vi "Configure Specific Limit Test.vi"(0 "VISA resource name":refnum<visa-resource-name>, 1 "Enable Limit Test  (T:Enable)":bool=TRUE, 5 "Limit Test Number (2)":u16=2, 7 "Low Limit (0)":dbl, 9 "High Limit (1)":dbl=1.0, 11 "error in (no error)":errorcluster, 12 "I/O Output Settings":T1) -> (4 "VISA resource name out":refnum<visa-resource-name>, 15 "error out":errorcluster)   [LabVIEW 2015, in "VIPM2.lvlib" / "Keithley 24XX.lvlib"]
doc: "Configures limit testing settings, such as the source of the tested value, binning, and I/O settings."
uses:
  Keithley 24XX.lvlib
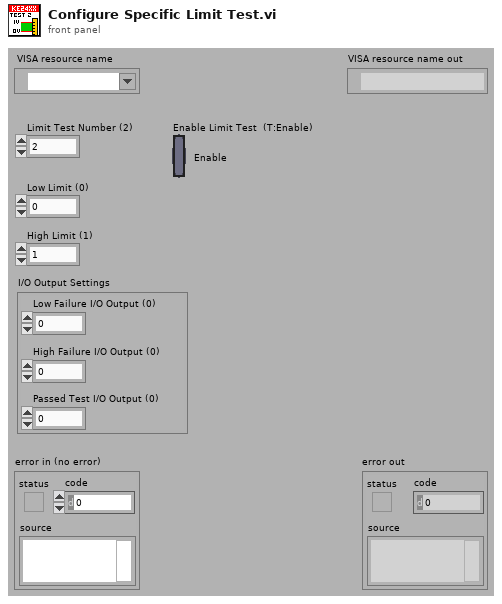
[diagram p1: front panel]
types:
  T1 = cluster{"Low Failure I/O Output (0)":dbl, "High Failure I/O Output (0)":dbl, "Passed Test I/O Output (0)":dbl}
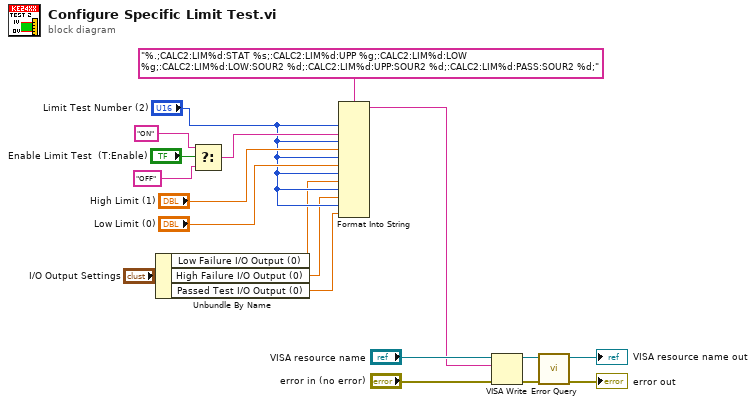
[diagram p0: block diagram]
diagram:
  n1 = Unbundle By Name("I/O Output Settings") -> ("Low Failure I/O Output (0)"=w5:dbl, "High Failure I/O Output (0)"=w4:dbl, "Passed Test I/O Output (0)"=w3:dbl)
  n2 = Select(t="ON", s="Enable Limit Test  (T:Enable)", f="OFF") -> (s? t:f=w10:string)
  n3 = Format Into String(format string="%.;CALC2:LIM%d:STAT %s;:CALC2:LIM%d:UPP %g;:CALC2:LIM%d:LOW %g;:CALC2:LIM%d:LOW:SOUR2 %d;:CALC2:LIM%d:UPP:SOUR2 %d;:CALC2:LIM%d:PASS:SOUR2 %d;", "Limit Test Number (2)", w10, "Limit Test Number (2)", "High Limit (1)", "Limit Test Number (2)", "Low Limit (0)", "Limit Test Number (2)", w5, "Limit Test Number (2)", w4, "Limit Test Number (2)", w3) -> (resulting string=w1:string)  [unwired: 2 in, 1 out]
  n4 = VISA Write(VISA resource name="VISA resource name", write buffer=w1, error in (no error)="error in (no error)") -> (VISA resource name out=w15:refnum<visa-resource-name>, error out=w14:errorcluster)  [unwired: 1 out]
  n5 = call "Error Query.vi"("error in (no error)"=w14, "VISA resource name"=w15) -> ("error out"=→"error out":errorcluster, "VISA resource name out"=→"VISA resource name out":refnum<visa-resource-name>)  [unwired: 6 in, 2 out]
